vi "Testing Info Folder.vi"() -> ()   [LabVIEW 2013]
panel:
  out "New":path
  out "Current VI":path
  out "Get File Foldre Path":path
  in  "stop":bool
  out "Info Folder":path
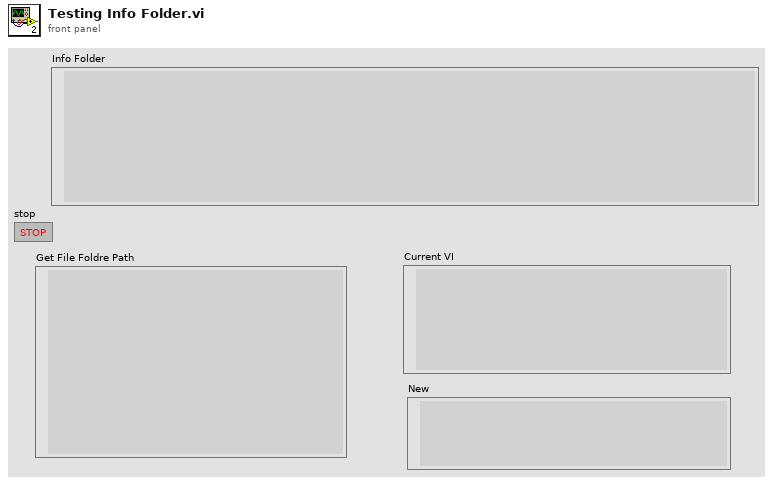
[diagram p1: front panel]
types:
  T1 = enum32{"invalid app kind", "Development System", "Run Time System", "Student Edition", "Embedded LabVIEW", "Evaluation", "Custom"}
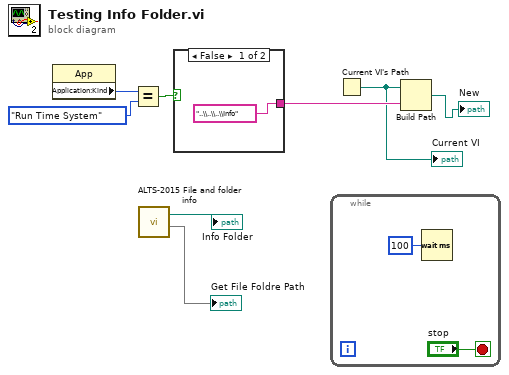
[diagram p0: block diagram]
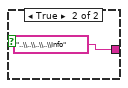
[diagram p2: hidden frame]
diagram:
  n1 = property class="App"() -> ("Application:Kind"=w6:T1)  [unwired: 2 in, 2 out]
  n2 = Equal?(x=w6, y=T1."Run Time System") -> (x = y?=w4:bool)
  n3 = call "ALTS-2015 File and folder info.vi"() -> ("Info Folder"=→"Info Folder":path, 9:→"Get File Foldre Path")  [unwired: 2 in, 8 out]
  n4 = case shown="False" w4 {
    tunnel: ["..\\..\\..\\Info" ("name or relative path") "..\\..\\..\\..\\Info" ("name or relative path")] -> w3
    frame False {
    }
    frame True {
    }
  }
  n5 = while {
    stop <- "stop" stop-if-true
    n6 = Wait (ms)(milliseconds to wait=u32 100) -> ()  [unwired: 1 out]
  }
  n7 = Current VI's Path() -> (path=w2:path)
  "Current VI" <- w2
  n8 = Build Path(base path=w2, name or relative path=w3) -> (appended path=→"New":path)
